vi "Log_pression_vessie.vi"(0 "LogFilePath":path) -> ()   [LabVIEW 2019]
panel:
  in  "Numérique 3":dbl
  in  "Numérique 2":dbl
  in  "Numérique":dbl
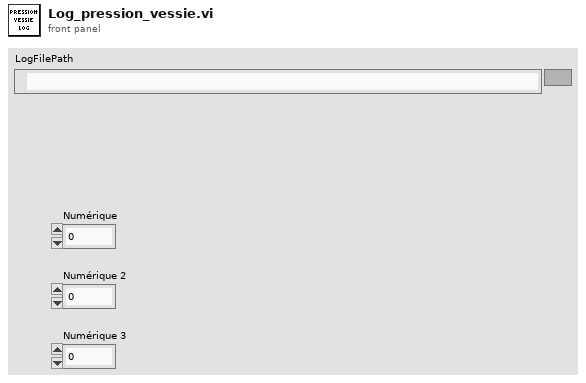
[diagram p1: front panel]
types:
  T1 = enum16{"open", "replace", "create", "open or create", "replace or create", "replace or create with confirmation"}
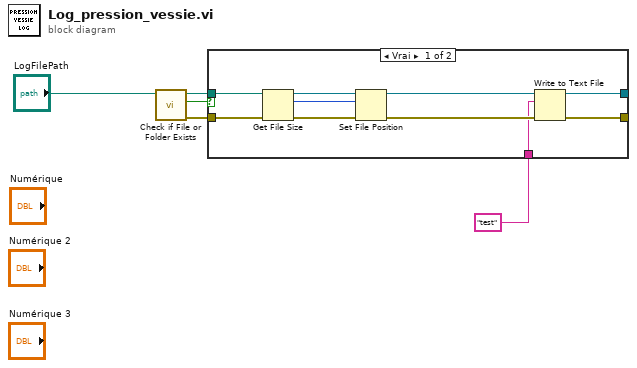
[diagram p0: block diagram]
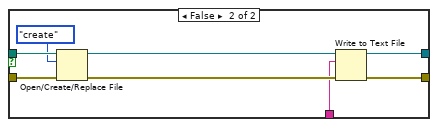
[diagram p2: hidden frame]
diagram:
  n1 = call <vilib>:"Check if File or Folder Exists.vi"("path"="LogFilePath") -> ("error out"=w2:errorcluster, "file or folder exists?"=w4:bool, "dup path"=w3:path)  [unwired: 8 in]
  n2 = case shown="Vrai" w4 {
    tunnel: w3 -> [w10 w23]
    tunnel: w2 -> [w9 w22]
    tunnel: [w15 w21] -> _
    tunnel: [w14 w20] -> _
    tunnel: "test" ("texte") -> [w6 w16]
    frame True {
      n3 = Get File Size(file=w10, error in=w9) -> (refnum out=w13:refnum<file>, size (in bytes)=w12:i64, 0:w11:errorcluster)
      n4 = Set File Position(offset (in bytes) (0)=w12, refnum=w13, error in=w11) -> (refnum out=w8:refnum<file>, error out=w7:errorcluster)  [unwired: 1 in]
      n5 = Write to Text File(file (use dialog)=w8, text=w6, error in=w7) -> (refnum out=w15:refnum<file>, error out=w14:errorcluster)  [unwired: 1 in, 1 out]
    }
    frame False {
      n6 = Open/Create/Replace File(file path (use dialog)=w23, error in=w22, operation (0:open)=T1."create") -> (refnum out=w18:refnum<file>, error out=w17:errorcluster)  [unwired: 3 in, 1 out]
      n7 = Write to Text File(file (use dialog)=w18, text=w16, error in=w17) -> (refnum out=w21:refnum<file>, error out=w20:errorcluster)  [unwired: 1 in, 1 out]
    }
  }
